vi "sample8(BlockR All).vi"() -> ()   [LabVIEW 2011]
uses:
  <vilib>/Platform/TimedLoop/XDataNode/timing_clust.ctl
  <vilib>/Platform/TimedLoop/XDataNode/nitl_modes.ctl
  <vilib>/Platform/TimedLoop/XDataNode/wakeup.ctl
  <vilib>/Platform/TimedLoop/XDataNode/XDataNode.xnode
  <vilib>/Platform/TimedLoop/XDataNode/XDNodeRunTimeDep.lvlib
panel:
  out "Name/ModelNo":u16(ring)=350 items=["XL320"=350, "H54-200-S500-R"=54024, "H54-100-S500-R"=53768, "H42-20-S300-R"=51200, "M54-60-S250-R"=46352, "M54-40-S250-R"=46096, "M42-10-S260-R"=43288, "L54-50-S290-R"=38176, "L54-50-S500-R"=38152, "L54-30-S400-R"=37928, "L54-30-S500-R"=37896, "L42-10-S300-R"=35072, "XL430-W250"=1060, "XM430-W210"=1030, "XH430-W210"=1010, "XM430-V210"=1050, "XM430-W350"=1020, "XH430-W350"=1000, "XM430-V350"=1040, "MX-28"=30, "MX-64"=311, "MX-106"=321]
  out "err":errorcluster caption="エラー出力" {"code" format="%04x"}
  out "present load":i16
  in  "UPDATE":bool
  out "ACK":bool
  in  "TorqueEnable":bool
  in  "OffsetTime":u32=20
  in  "frequency":dbl=0.2 min=0.0 max=10.0 step=0.05
  in  "waveform":enum16{"sin", "square"}(ring)
  in  "Target ID":u8=1 max=253
  in  "Baudrate":u32=1000000 min=9600 max=3000000 step=100
  in  "COM":refnum<visa-resource-name> caption="COMポート"
  in  "wave":bool
  out "CtrlTable":u8[](array[numeric]) format="%02x"
  out "Chart":T1(graph)
  out "STOP2":bool
  out "present position":i32
  in  "STOP":bool
  in  "goal position":i32(knob)
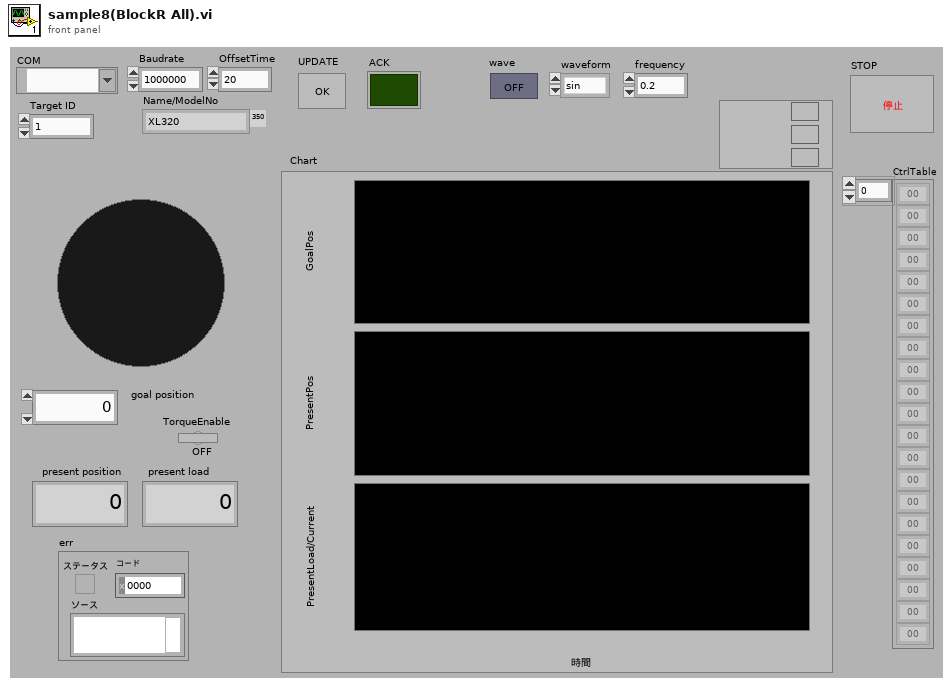
[diagram p1: front panel]
types:
  T1 = cluster{"goal position":i32, "present position":i32, "present load":i16}
  T2 = typedef "XDNodeRunTimeDep.lvlib/timing_clust.ctl" = cluster{"Expected End [f-1]":u64, "Actual End [f-1]":u64, "Finished Late? [f-1]":bool, "Expected End [i-1]":u64, "Actual End [i-1]":u64, "Finished Late? [i-1]":bool, "Expected Start [i]":u64, "Actual Start [i]":u64, "Expected Start [f]":u64, "Actual Start [f]":u64, "Source Name":string, "Structure Name":string, "Period":i64, "Deadline":i64, "Offset":i64, "Start":i64, "Priority":i32, "Timeout":i32, "Mode":T3, "Wakeup Reason":T4, "Error":errorcluster, "Source Type":string, "Secondary Source Type":string, "Global End Time":u64, "Global Start Time":u64, "Frame Duration":u64, "Iteration Duration":u64, "Assigned CPU":i32, "I/O Scan Engine Mode":u32}
  T3 = typedef "XDNodeRunTimeDep.lvlib/nitl_modes.ctl" = enum32{"No Change", "Process missed periods, maintain original phase", "Discard missed periods, maintain original phase", "Process missed periods, ignore original phase", "Discard missed periods, ignore original phase"}
  T4 = typedef "XDNodeRunTimeDep.lvlib/wakeup.ctl" = enum32{"Normal", "Aborted", "Asynchronous wakeup", "Timing source error", "Timed loop error", "Timeout"}
  T5 = cluster{"Name/ModelNo":u16, "Type":u8, "MaxPosition":i32, "MinPosition":i32, "ScaleFactor":dbl}
  T6 = cluster{"ACK":bool, "ID":u8, "MaxPositionLimit":cluster{"address":u16, "width":u8, "limit":cluster{"max":i32, "min":i32}}, "MinPositionLimit":cluster{"address":u16, "width":u8, "limit":cluster{"max":i32, "min":i32}}, "TorqueEnable":cluster{"address":u16, "width":u8, "limit":cluster{"max":i32, "min":i32}}, "GoalPosition":cluster{"address":u16, "width":u8, "limit":cluster{"max":i32, "min":i32}}, "GoalVelocity":cluster{"address":u16, "width":u8, "limit":cluster{"max":i32, "min":i32}}, "PresentPosition":cluster{"address":u16, "width":u8, "limit":cluster{"max":i32, "min":i32}}, "PresentVelocity":cluster{"address":u16, "width":u8, "limit":cluster{"max":i32, "min":i32}}, "HardwareError":cluster{"address":u16, "width":u8, "limit":cluster{"max":i32, "min":i32}}}
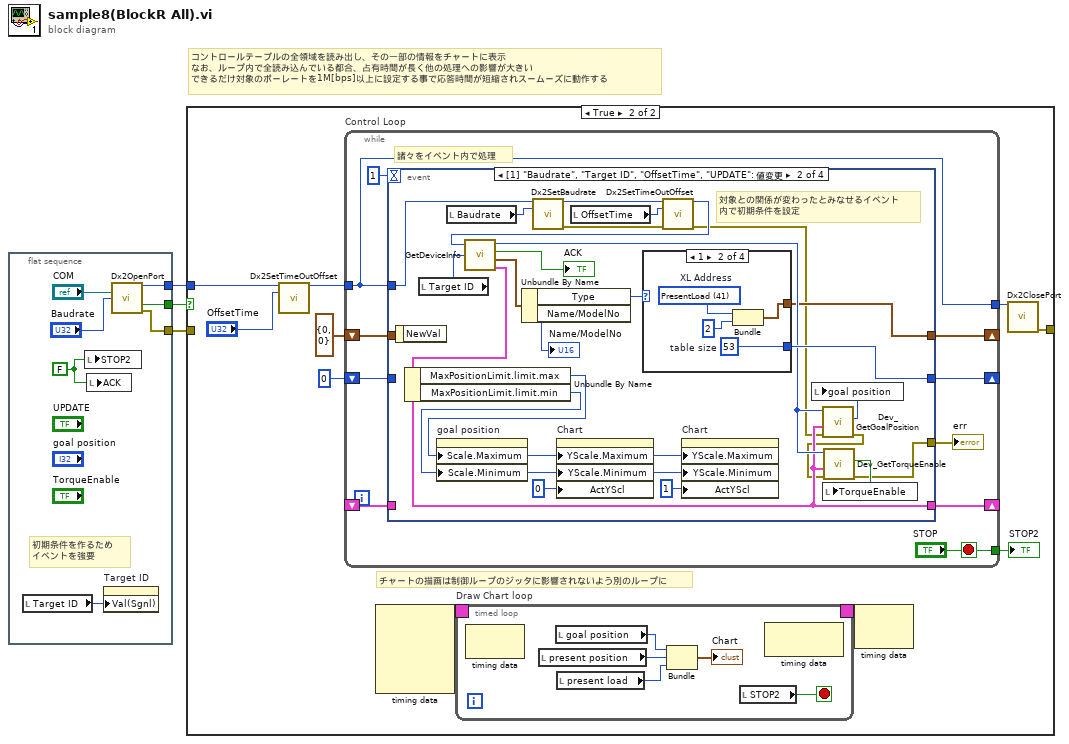
[diagram p0: block diagram]
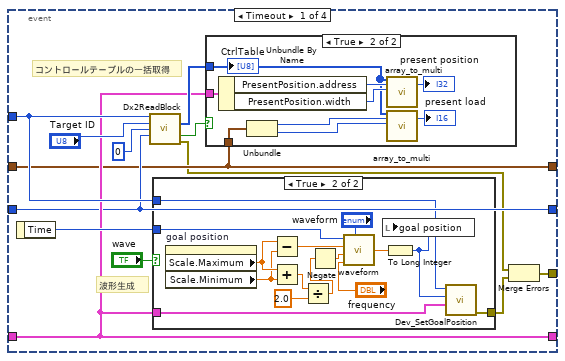
[diagram p3: hidden frame]
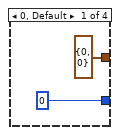
[diagram p6: hidden frame]
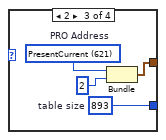
[diagram p7: hidden frame]
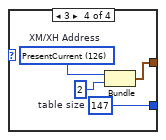
[diagram p8: hidden frame]
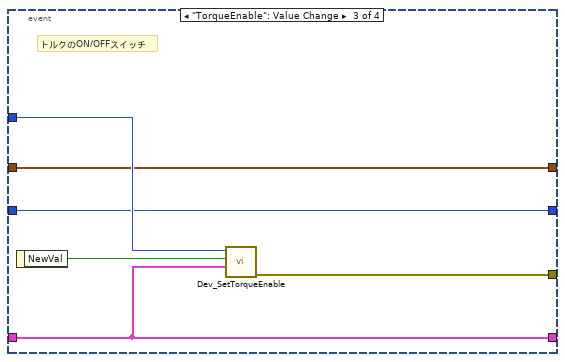
[diagram p9: hidden frame]
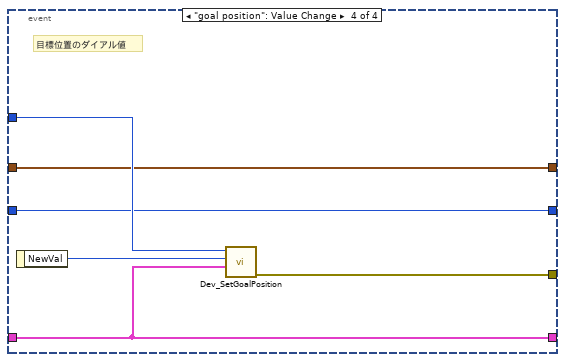
[diagram p10: hidden frame]
diagram:
  # "コントロールテーブルの全領域を読み出し、その一部の情報をチャートに表示\nなお、ループ内で全読み込んでいる都合、占有時間が長く他の処理への影響が大きい\nできるだけ対象のボーレートを1M[bps]以上に設定する事で応答時間が短縮されスームーズに動作する"
  n1 = flat-sequence {
    tunnel: [w10] -> w3
    tunnel: [w9] -> w2
    tunnel: [w8] -> w1
    frame #0 {
      w5 = FALSE ("停止 3")
      # "初期条件を作るため\nイベントを強要"
      n2 = local read "Target ID"() -> (w4:u8)
      n3 = local write "STOP2"(w5) -> ()
      n4 = local write "ACK"(w5) -> ()
      n5 = property on="Target ID" class="DigNum （指定）"("Val(Sgnl)"=w4) -> ()  [unwired: 2 in, 2 out]
      n6 = call "Dx2OpenPort.vi"("port"="COM", "baudrate"="Baudrate") -> ("dvid"=w9:u32, "成功"=w8:bool, "エラー出力"=w10:errorcluster)  [unwired: 11 in]
    }
  }
  n7 = case shown="TRUE" w1 {
    tunnel: w3 -> [w11 _]
    tunnel: w2 -> [_ w17]
    tunnel: [w11 w19] -> _
    frame False {
    }
    frame True {
      # "チャートの描画は制御ループのジッタに影響されないよう別のループに"
      n8 = call "Dx2SetTimeOutOffset.vi"("dvid in"=w17, "OffsetTime"="OffsetTime") -> ("dvid out"=w15:u32)  [unwired: 12 in, 1 out]
      n9 = while "Control Loop" {
        shift-right: [w31] -> _
        shift-left: _ -> [w30]
        shift-right: [w29] -> _
        shift-left: u32 0 ("size") -> [w28]
        tunnel: w15 -> [w25]
        tunnel: ["STOP"] -> w16
        tunnel: [w25] -> w14
        shift-right: [w24] -> _
        shift-left: cluster{"XM/XM Address":u16, u8} {"XM/XM Address"=0, 0} -> [w23]
        stop <- "STOP" stop-if-true
        # "諸々をイベント内で処理"
        n10 = event shown="[1] \"Baudrate\", \"Target ID\", \"OffsetTime\", \"UPDATE\": 値変更" {
          selector: _ -> [_ _ _ _]
          dyn-events: _ -> [_ _ _ _]
          timeout: 1 -> [_ _ _ _]
          tunnel: [w37 w77 w110 w116] -> w31
          tunnel: w30 -> [w37 _ w110 w116]
          tunnel: [w34 w70 w107 w113] -> w22
          tunnel: [w36 w83 w109 w115] -> w29
          tunnel: w25 -> [w39 w82 w112 w117]
          tunnel: w28 -> [w36 _ w109 w115]
          tunnel: [w35 w78 w108 w114] -> w24
          tunnel: w23 -> [w35 _ w108 w114]
          event Timeout {
            # "波形生成"
            # "コントロールテーブルの一括取得"
            n11 = event-data() -> ("Time"=w40:u32)  [unwired: 1 in]
            n12 = call "Dx2ReadBlock.vi"("dvid in"=w39, "id"="Target ID", "address"=u16 0, "size"=w36) -> ("data out"=w43:u8[], "成功"=w42:bool, "エラー出力"=w32:errorcluster)  [unwired: 8 in, 1 out]
            n13 = case shown="TRUE" "wave" {
              tunnel: w37 -> [_ w59]
              tunnel: w40 -> [_ w58]
              tunnel: w39 -> [_ w56]
              tunnel: [_ w55] -> w33
              frame False {
              }
              frame True {
                n14 = property on="goal position" class="Knob （指定）"() -> ("Scale.Maximum"=w51:dbl, "Scale.Minimum"=w50:dbl)  [unwired: 2 in, 2 out]
                n15 = Subtract(x=w51, y=w50) -> (x-y=w52:dbl)
                n16 = Add(x=w51, y=w50) -> (x+y=w49:dbl)
                n17 = Divide(x=w49, y=2.0) -> (x/y=w48:dbl)
                n18 = Negate(x=w48) -> (-x=w45:dbl)
                n19 = call "waveform.vi"("time(ms)"=w58, "amplitude"=w52, "offset"=w45, "frequency"="frequency", "waveform"="waveform") -> ("wave"=w57:dbl)
                n20 = To Long Integer(number=w57) -> (32bit integer=w46:i32)
                n21 = local write "goal position"(w46) -> ()
                n22 = call "Dev_SetGoalPosition.vi"("ItemInfo"=w59, "goal position"=w46, "dvid in"=w56) -> ("エラー出力"=w55:errorcluster)  [unwired: 2 in, 2 out]
              }
            }
            n23 = case shown="TRUE" w42 {
              tunnel: w43 -> [_ w63]
              tunnel: w37 -> [_ w65]
              tunnel: w35 -> [_ w60]
              frame False {
              }
              frame True {
                n24 = Unbundle By Name(w65) -> ("PresentPosition.address"=w68:u16, "PresentPosition.width"=w67:u8)
                n25 = Unbundle(w60) -> ("XM/XM Address"=w62:u16, w61:u8)
                n26 = call "array_to_multi.vi"("array"=w63, "OffsetAddr"=w68, "length"=w67) -> ("uint32"=→"present position":u32)  [unwired: 16 in]
                n27 = call "array_to_multi.vi"("array"=w63, "OffsetAddr"=w62, "length"=w61) -> ("uint32"=→"present load":u32)  [unwired: 16 in]
                "CtrlTable" <- w63
              }
            }
            n28 = Merge Errors(w32, w33) -> (w34:errorcluster)
          }
          event "Baudrate", "Target ID", "OffsetTime", "UPDATE": Value Change {
            # "対象との関係が変わったとみなせるイベント\n内で初期条件を設定"
            n29 = event-data() -> ()  [unwired: 1 in, 1 out]
            n30 = local read "Target ID"() -> (w86:u8)
            n31 = local read "Baudrate"() -> (w91:u32)
            n32 = call "Dx2SetBaudrate.vi"("dvid in"=w82, "Baudrate"=w91) -> ("dvid out"=w89:u32, "エラー出力"=w88:errorcluster)  [unwired: 11 in, 1 out]
            n33 = local read "OffsetTime"() -> (w90:u32)
            n34 = call "Dx2SetTimeOutOffset.vi"("dvid in"=w89, "OffsetTime"=w90, "エラー入力"=w88) -> ("dvid out"=w87:u32, "エラー出力"=w72:errorcluster)  [unwired: 11 in]
            n35 = call "GetDeviceInfo.vi"("dvid in"=w87, "Target ID"=w86) -> ("dvid out"=w81:u32, "matched"=→"ACK":bool, "TargetInfo"=w85:T5, "ItemInfo"=w77:T6)  [unwired: 1 in]
            n36 = Unbundle By Name(w77) -> ("MaxPositionLimit.limit.max"=w73:i32, "MaxPositionLimit.limit.min"=w74:i32)
            n37 = property on="goal position" class="Knob （指定）"("Scale.Maximum"=w73, "Scale.Minimum"=w74) -> ()  [unwired: 2 in, 2 out]
            n38 = Unbundle By Name(w85) -> ("Type"=w84:u8, "Name/ModelNo"=→"Name/ModelNo":u16)
            n39 = property on="Chart" class="WFChart （指定）"("YScale.Maximum"=w73, "YScale.Minimum"=w74, "ActYScl"=0 ("アクティブYスケール")) -> ()  [unwired: 2 in, 2 out]
            n40 = case shown="1" w84 {
              tunnel: [u32 0 ("size") w98 w102 w106] -> w83
              tunnel: [cluster{"XM/XM Address":u16, u8} {"XM/XM Address"=0, 0} w95 w99 w103] -> w78
              frame 0, Default {
              }
              frame 1 {
                w97 = u16 41 items=["ModelNo"=0, "VersionOfFirmware"=2, "ID"=3, "Baudrate"=4, "ReturnDelayTime"=5, "CWAngleLimit"=6, "CCWAngleLimit"=8, "ControlMode"=11, "LimitTemperature"=12, "LowestLimitVoltage"=13, "HighestLimitVoltage"=14, "MaxTorque"=15, "StatusReturnLevel"=17, "AlarmShutdown"=18, "TorqueEnable"=24, "LED"=25, "DGain"=26, "IGain"=27, "PGain"=28, "GoalPosition"=30, "GoalVelocity"=32, "GoalTorque"=35, "PresentPosition"=37, "PresentSPeed"=39, "PresentLoad"=41, "PresentVoltage"=45, "PresentTemperature"=46, "RegistedInstruction"=47, "Moving"=49, "HardwareErrorStatus"=50, "Punch"=51]  # XL Address
                w98 = u32 53  # table size
                n41 = Bundle("XL Address"=w97, u8 2) -> (w95:cluster{"XL Address":u16, u8})  [unwired: 1 in]
              }
              frame 2 {
                w100 = u16 621 items=["ModelNo"=0, "ModelInfo"=2, "VersionOfFirmware"=6, "ID"=7, "Baudrate"=8, "ReturnDelayTime"=9, "OperationMode"=11, "HormingOffset"=13, "MovingThreshold"=17, "TemperatureLimit"=21, "MaxVoltageLimit"=22, "MinVoltageLimit"=24, "AccelerationLimit"=26, "TorqueLimit"=30, "VoltageLimit"=32, "MaxPositionLimit"=36, "MinPositionLimit"=40, "ExternalPortMode1"=44, "ExternalPortMode2"=45, "ExternalPortMode3"=46, "ExternalPortMode4"=47, "Shutdown"=48, "TorqueEnable"=562, "LED_Red"=563, "LED_Green"=564, "LED_Blue"=565, "VelocityIGain"=586, "VelocityPGain"=588, "PositionPGain"=594, "GoalPosition"=596, "GoalVelocity"=600, "GoalTorque"=604, "GoalAcceleration"=606, "Moving"=610, "PresentPosition"=611, "PresentVelocity"=615, "PresentCurrent"=621, "PresentInputVoltage"=623, "PresentTemperature"=625, "ExternalPortData1"=626, "ExternalPortData2"=628, "ExternalPortData3"=630, "ExternalPortData4"=632, "RegistedInstruction"=890, "StatusReturnLevel"=891, "HardwareError"=892]  # PRO Address
                w102 = u32 893  # table size
                n42 = Bundle("PRO Address"=w100, u8 2) -> (w99:cluster{"PRO Address":u16, u8})  [unwired: 1 in]
              }
              frame 3 {
                w104 = u16 126 items=["ModelNo"=0, "ModelInfo"=2, "VersionOfFirmware"=6, "ID"=7, "Baudrate"=8, "ReturnDelayTime"=9, "OperationMode"=11, "ProtocolVersion"=13, "HormingOffset"=20, "MovingThreshold"=24, "TemperatureLimit"=31, "MaxVoltageLimit"=32, "MinVoltageLimit"=34, "PWMLimit"=36, "CurrentLimit"=38, "AccelerationLimit"=40, "VelocityLimit"=44, "MaxPositionLimit"=48, "MinPositionLimit"=52, "Shutdown"=63, "TorqueEnable"=64, "LED"=65, "StatusReturnLevel"=68, "RegistedInstruction"=69, "HardwareErrorStatus"=70, "VelocityIGain"=76, "VelocityPGain"=78, "VelocityDGain"=80, "PositionIGain"=82, "PositionPGain"=84, "FeedForward2ndGain"=88, "FeedForward1stGain"=90, "GoalPWM"=100, "GoalCurrent"=102, "GoalVelocity"=104, "ProfileAcceleration"=108, "ProfileVelocity"=112, "GoalPosition"=116, "RealtimeTick"=120, "Moving"=122, "MovingStatus"=123, "PresentPWM"=124, "PresentCurrent"=126, "Presentvelocity"=128, "PresentPosition"=132, "VelocityTrajectory"=136, "PositionTrajectory"=140, "PresentIInputVoltage"=144, "PresentTemperature"=146]  # XM/XH Address
                w106 = u32 147  # table size
                n43 = Bundle("XM/XH Address"=w104, u8 2) -> (w103:cluster{"XM/XH Address":u16, u8})  [unwired: 1 in]
              }
            }
            n44 = property on="Chart" class="WFChart （指定）"("YScale.Maximum"=w73, "YScale.Minimum"=w74, "ActYScl"=1 ("アクティブYスケール")) -> ()  [unwired: 2 in, 2 out]
            n45 = call "Dev_GetGoalPosition.vi"("エラー入力"=w72, "ItemInfo"=w77, "dvid in"=w81) -> ("エラー出力"=w71:errorcluster, "goal position"=w80:i32)  [unwired: 1 in, 2 out]
            n46 = local write "goal position"(w80) -> ()
            n47 = call "Dev_GetTorqueEnable.vi"("エラー入力"=w71, "ItemInfo"=w77, "dvid in"=w81) -> ("エラー出力"=w70:errorcluster, "torque enable"=w79:bool)  [unwired: 1 in, 2 out]
            n48 = local write "TorqueEnable"(w79) -> ()
          }
          event "TorqueEnable": Value Change {
            # "トルクのON/OFFスイッチ"
            n49 = event-data() -> ("NewVal"=w111:bool)  [unwired: 1 in]
            n50 = call "Dev_SetTorqueEnable.vi"("ItemInfo"=w110, "torque enable"=w111, "dvid in"=w112) -> ("エラー出力"=w107:errorcluster)  [unwired: 2 in, 2 out]
          }
          event "goal position": Value Change {
            # "目標位置のダイアル値"
            n51 = event-data() -> ("NewVal"=w118:i32)  [unwired: 1 in]
            n52 = call "Dev_SetGoalPosition.vi"("ItemInfo"=w116, "goal position"=w118, "dvid in"=w117) -> ("エラー出力"=w113:errorcluster)  [unwired: 2 in, 2 out]
          }
        }
        "err" <- w22
      }
      "STOP2" <- w16
      n53 = node-c288() -> (w21:T2)  [unwired: 4 in]
      n54 = timed-loop "Draw Chart loop" {
        timing: w21 -> [_]
        timing-out: [_] -> w20
        stop <- w123 stop-if-true
        n55 = node-c288() -> ()  [unwired: 1 in, 1 out]
        n56 = local read "present position"() -> (w121:i32)
        n57 = local read "goal position"() -> (w122:i32)
        n58 = local read "present load"() -> (w119:i16)
        n59 = Bundle("goal position"=w122, "present position"=w121, "present load"=w119) -> (→"Chart":T1)  [unwired: 1 in]
        n60 = local read "STOP2"() -> (w123:bool)
        n61 = node-c288() -> ()  [unwired: 1 in, 1 out]
      }
      n62 = node-c288(w20) -> ()  [unwired: 1 out]
      n63 = call "Dx2ClosePort.vi"("dvid"=w14) -> ("エラー出力"=w19:errorcluster)  [unwired: 13 in, 1 out]
    }
  }
